vi "Dialog.MassStepGeneration.vi"(8 "error in (no error)":errorcluster, 11 "Cluster":T1) -> (0 "error out":errorcluster)   [LabVIEW 2013, in "Simple Sequence Editor.lvlib"]
uses:
  Simple Sequence Editor.lvlib
  Types/StateVariables.ctl
  Types/ChannelProperties.ctl
panel:
  in  "Cancel":bool
  in  "OK":bool
  in  "Starting Step Index":u16 max=0
  in  "Value Increment":dbl
  in  "# of Step":u16=1
  in  "Base Step":string(combo)="Step (Value)"
  in  "Alias":string(combo)
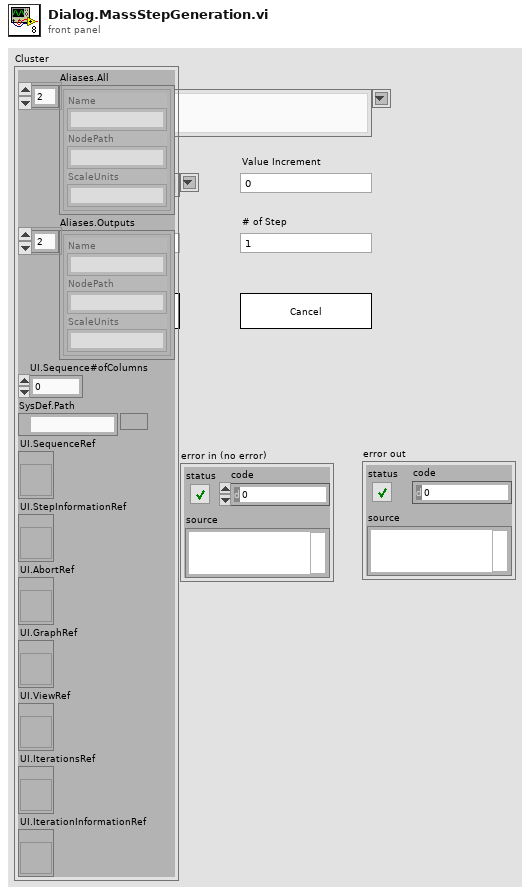
[diagram p1: front panel]
types:
  T1 = typedef "Simple Sequence Editor.lvlib/StateVariables.ctl" = cluster{"Aliases.All":T2[], "Aliases.Outputs":T2[], "UI.Sequence#ofColumns":i32, "SysDef.Path":path, "UI.SequenceRef":refnum<vi>, "UI.StepInformationRef":refnum<vi>, "UI.AbortRef":refnum<vi>, "UI.GraphRef":refnum<vi>, "UI.ViewRef":refnum<vi>, "UI.IterationsRef":refnum<vi>, "UI.IterationInformationRef":refnum<vi>}
  T2 = typedef "Simple Sequence Editor.lvlib/ChannelProperties.ctl" = cluster{"Name":string, "NodePath":string, "ScaleUnits":string}
  T3 = enum8{"Enabled", "Disabled", "Disabled and Grayed Out"}
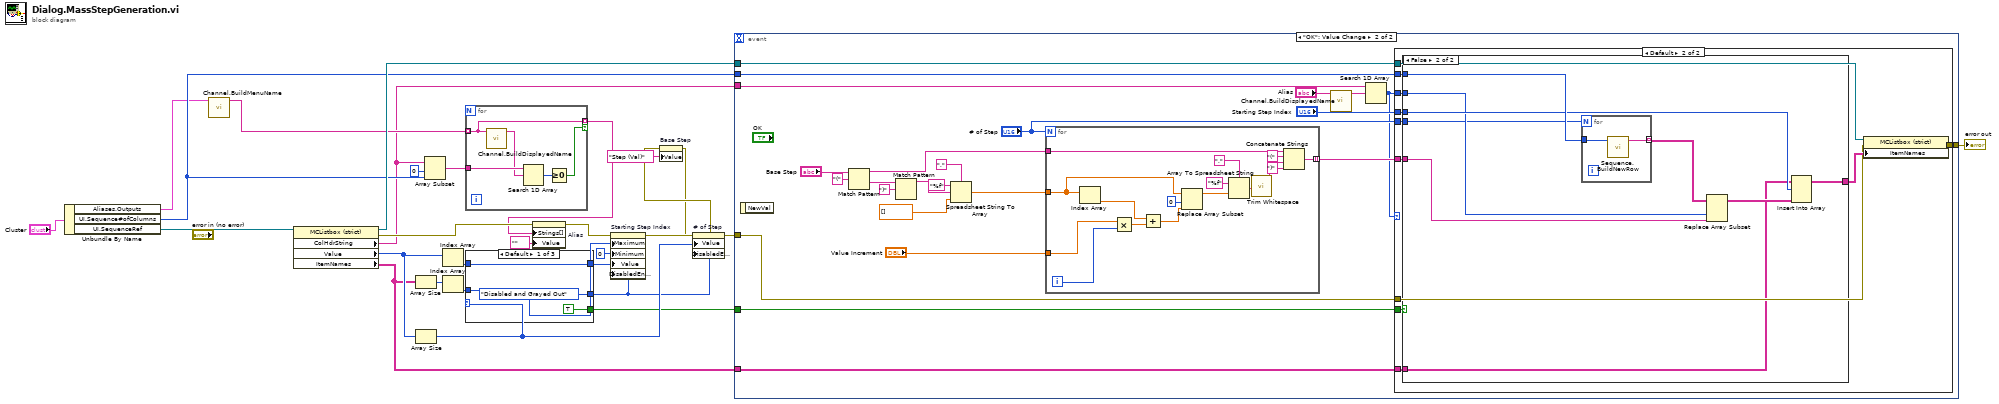
[diagram p0: block diagram]
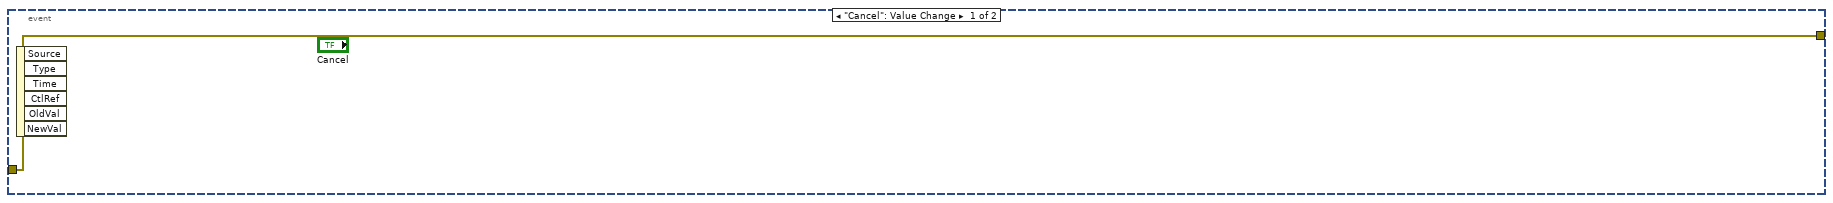
[diagram p2: hidden frame]
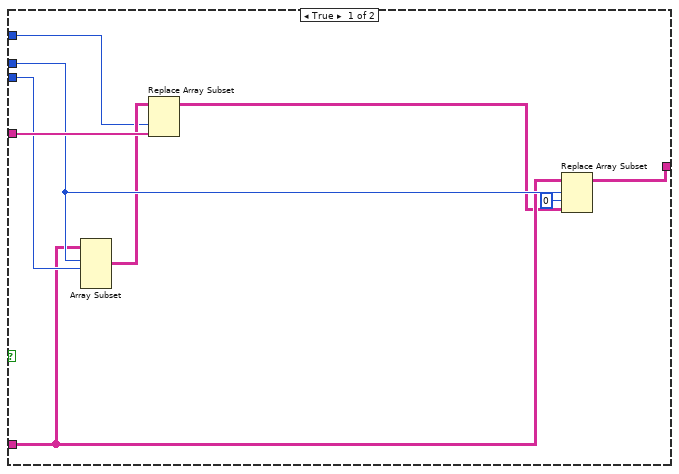
[diagram p4: hidden frame]
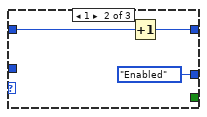
[diagram p5: hidden frame]
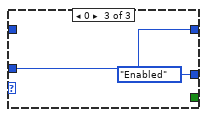
[diagram p6: hidden frame]
diagram:
  n1 = Unbundle By Name("Cluster") -> ("Aliases.Outputs"=w9:T2[], "UI.Sequence#ofColumns"=w17:i32, "UI.SequenceRef"=w27:refnum<vi>)
  n2 = call "Channel.BuildMenuName.vi"("Aliases"=w9) -> ("Aliases Array"=w8:string[])  [unwired: 10 in]
  n3 = property class="MCListbox (strict)"(reference=w27) -> (reference out=w19:refnum<vi>, error out=w15:errorcluster, "ColHdrString"=w7:string[], "Value"=w21:i32[], "ItemNames"=w20:string[][])  [unwired: 1 in]
  n4 = Array Size(array=w20) -> (size(s)=w25:i32[])
  n5 = Array Size(array=w21) -> (size(s)=w13:i32)
  n6 = Array Subset(array=w7, index=0, length=w17) -> (w6:string[])
  n7 = Index Array(array=w21) -> (element=w26:i32)  [unwired: 1 in]
  n8 = Index Array(array=w25) -> (element=w24:i32)  [unwired: 1 in]
  n9 = for {
    tunnel: w8 -> [w31] mode=indexing
    tunnel: w6 -> [w33]
    tunnel: [w31] -> w5 mode=indexing if=w29
    n10 = call "Channel.BuildDisplayedName.vi"("Path"=w31) -> ("Formated Path"=w32:string)  [unwired: 10 in]
    n11 = Search 1D Array(1D array=w33, element=w32) -> (index of element=w30:i32)  [unwired: 1 in]
    n12 = Greater Or Equal To 0?(x=w30) -> (x >= 0?=w29:bool)
  }
  n13 = case shown="Default" w13 {
    tunnel: [w36 w38 w41] -> w22
    tunnel: w26 -> [w36 w39 _]
    tunnel: w24 -> [_ _ w41]
    tunnel: [T3."Disabled and Grayed Out" ("Disabled") T3."Enabled" ("Disabled") T3."Enabled" ("Disabled")] -> w11
    tunnel: [TRUE _ _] -> w10
    frame Default {
    }
    frame 1 {
      n14 = Increment(x=w39) -> (x+1=w38:i32)
    }
    frame 0 {
    }
  }
  n15 = property on="Alias" class="CmbBox"(error in=w15, "Strings[]"=w5, "Value"="" ("Alias")) -> (error out=w14:errorcluster)  [unwired: 1 in, 1 out]
  n16 = property on="Starting Step Index" class="DigNum (strict)"(error in=w14, "Maximum"=w24, "Minimum"=0, "Value"=w22, "DisabledEnum"=w11) -> (error out=w12:errorcluster)  [unwired: 1 in, 1 out]
  n17 = property on="# of Step" class="DigNum (strict)"(error in=w12, "Value"=w13, "DisabledEnum"=w11) -> (error out=w2:errorcluster)  [unwired: 1 in, 1 out]
  n18 = property on="Base Step" class="CmbBox"(error in=w2, "Value"="Step (Val)" ("Base Step")) -> (error out=w1:errorcluster)  [unwired: 1 in, 1 out]
  n19 = event shown="[1] \"OK\": Value Change" {
    selector: _ -> [_ _]
    dyn-events: _ -> [_ _]
    timeout: _ -> [_ _]
    tunnel: w1 -> [w42 w46]
    tunnel: w7 -> [_ w54]
    tunnel: w20 -> [_ w51]
    tunnel: w17 -> [_ w52]
    tunnel: w19 -> [_ w48]
    tunnel: [w42 w45] -> w18
    tunnel: w10 -> [_ w44]
    event "Cancel": Value Change {
      n20 = event-data() -> ()  [unwired: 1 in, 6 out]
    }
    event "OK": Value Change {
      n21 = event-data() -> ()  [unwired: 1 in, 1 out]
      n22 = Match Pattern(string="Base Step", regular expression="(") -> (before substring=w56:string, after substring=w64:string)  [unwired: 1 in, 2 out]
      n23 = Match Pattern(string=w64, regular expression=")") -> (before substring=w62:string)  [unwired: 1 in, 3 out]
      n24 = Spreadsheet String To Array(delimiter (Tab)=",", format string="%f", spreadsheet string=w62, array type (2D Dbl)=dbl[] []) -> (array=w58:dbl[])
      n25 = for {
        N: "# of Step" -> [_]
        tunnel: w58 -> [w110]
        tunnel: "Value Increment" -> [w114]
        tunnel: w56 -> [w104]
        tunnel: [w100] -> w47 mode=indexing
        i -> [w113]
        n26 = Index Array(array=w110) -> (element=w111:dbl)  [unwired: 1 in]
        n27 = Multiply(x=w114, y=w113) -> (x*y=w112:dbl)
        n28 = Add(x=w111, y=w112) -> (x+y=w108:dbl)
        n29 = Replace Array Subset(array=w110, new element=w108, index=0) -> (w107:dbl[])
        n30 = Array To Spreadsheet String(delimiter (Tab)=",", array=w107, 3:"%f" ("format string")) -> (spreadsheet string=w102:string)
        n31 = call <vilib>:"Trim Whitespace.vi"("string"=w102) -> ("trimmed string"=w99:string)  [unwired: 1 in]
        n32 = Concatenate Strings(w104, "(" ("string"), w99, ")" ("string")) -> (w100:string)
      }
      n33 = call "Channel.BuildDisplayedName.vi"("Path"="Alias") -> ("Formated Path"=w53:string)  [unwired: 10 in]
      n34 = Search 1D Array(1D array=w54, element=w53) -> (index of element=w43:i32)  [unwired: 1 in]
      n35 = case shown="Default" w43 {
        tunnel: w52 -> [_ w78]
        tunnel: w51 -> [_ w77]
        tunnel: "# of Step" -> [_ w76]
        tunnel: "Starting Step Index" -> [_ w75]
        tunnel: w48 -> [_ w73]
        tunnel: w43 -> [_ w72]
        tunnel: w47 -> [_ w71]
        tunnel: w46 -> [w67 w70]
        tunnel: [w67 w69] -> w45
        tunnel: w44 -> [_ w68]
        frame -1 {
        }
        frame Default {
          n36 = case shown="False" w68 {
            tunnel: w78 -> [_ w96]
            tunnel: w77 -> [w82 w88]
            tunnel: w76 -> [w84 w91]
            tunnel: w75 -> [w85 w95]
            tunnel: [w87 w94] -> w74
            tunnel: w72 -> [w80 w92]
            tunnel: w71 -> [w86 w89]
            frame True {
              n37 = Array Subset(array=w82, index (row)=w85, length (row)=w84) -> (w83:string[][])  [unwired: 2 in]
              n38 = Replace Array Subset(array=w83, new element=w86, index (col)=w80) -> (w81:string[][])  [unwired: 1 in]
              n39 = Replace Array Subset(array=w82, new element=w81, index (row)=w85, index (col)=0 ("disabled index (col)")) -> (w87:string[][])
            }
            frame False {
              n40 = for {
                N: w91 -> [_]
                tunnel: w96 -> [w98]
                tunnel: [w97] -> w90 mode=indexing
                n41 = call "Sequence.BuildNewRow.vi"("UI.Sequence#ofColumns"=w98) -> ("New Array"=w97:string[])  [unwired: 10 in]
              }
              n42 = Replace Array Subset(array=w90, new element=w89, index (col)=w92) -> (w93:string[][])  [unwired: 1 in]
              n43 = Insert Into Array(array=w88, index (row)=w95, new element=w93) -> (w94:string[][])  [unwired: 1 in]
            }
          }
          n44 = property class="MCListbox (strict)"(reference=w73, error in=w70, "ItemNames"=w74) -> (error out=w69:errorcluster)  [unwired: 1 out]
        }
      }
    }
  }
  "error out" <- w18
